vi "Get Virtual Ports.vi"(8 "error in (no error)":errorcluster) -> (0 "error out":errorcluster, 3 "Serial Ports out":string[](array[string]))   [LabVIEW 2019, in "Listener.lvclass"]
uses:
  Listener.lvclass
  <vilib>/Utility/error.llb/whitespace.ctl
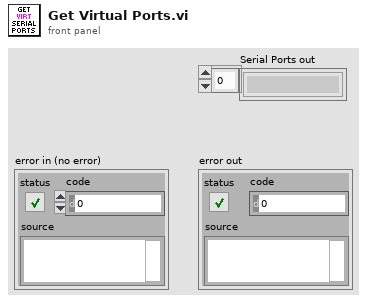
[diagram p1: front panel]
types:
  T1 = typedef "whitespace.ctl" = u16
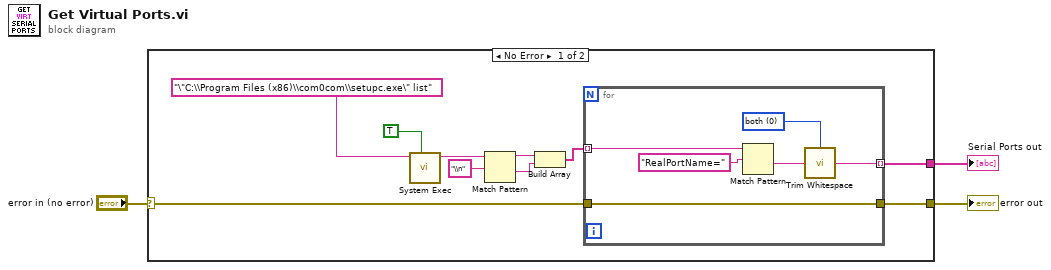
[diagram p0: block diagram]
diagram:
  n1 = case shown="No Error" "error in (no error)" {
    selector: "error in (no error)" -> [w6 w20]
    tunnel: [w5 w20] -> w3
    tunnel: [w4 _] -> w1
    frame No Error {
      n2 = call <vilib>:"System Exec.vi"("wait until completion? (T)"=TRUE, "command line"="\"C:\\Program Files (x86)\\com0com\\setupc.exe\" list") -> ("standard output"=w13:string)  [unwired: 6 in, 3 out]
      n3 = Match Pattern(string=w13, regular expression="\\n") -> (before substring=w12:string, after substring=w11:string)  [unwired: 1 in, 2 out]
      n4 = Build Array(w12, w11) -> (w7:string[])
      n5 = for {
        tunnel: w7 -> [w19] mode=indexing
        tunnel: w6 -> [w16]
        tunnel: [w16] -> w5
        tunnel: [w15] -> w4 mode=indexing
        w14 = T1 0 items=["both", "start of string", "end of string"] ("location (both)")
        n6 = Match Pattern(string=w19, regular expression="RealPortName=") -> (after substring=w17:string)  [unwired: 1 in, 3 out]
        n7 = call <vilib>:"Trim Whitespace.vi"("string"=w17, "location (both)"=w14) -> ("trimmed string"=w15:string)
      }
    }
    frame Error {
    }
  }
  "error out" <- w3
  "Serial Ports out" <- w1
